vi "Configure VIs for Development.vi"   [LabVIEW 2017]
types:
  T1 = cluster{"Status Message":refnum<data-value>, "Progress":refnum<data-value>, "Stop":refnum<data-value>}
  T2 = enum16{"Share clones between instances", "Preallocate clone for each instance"}
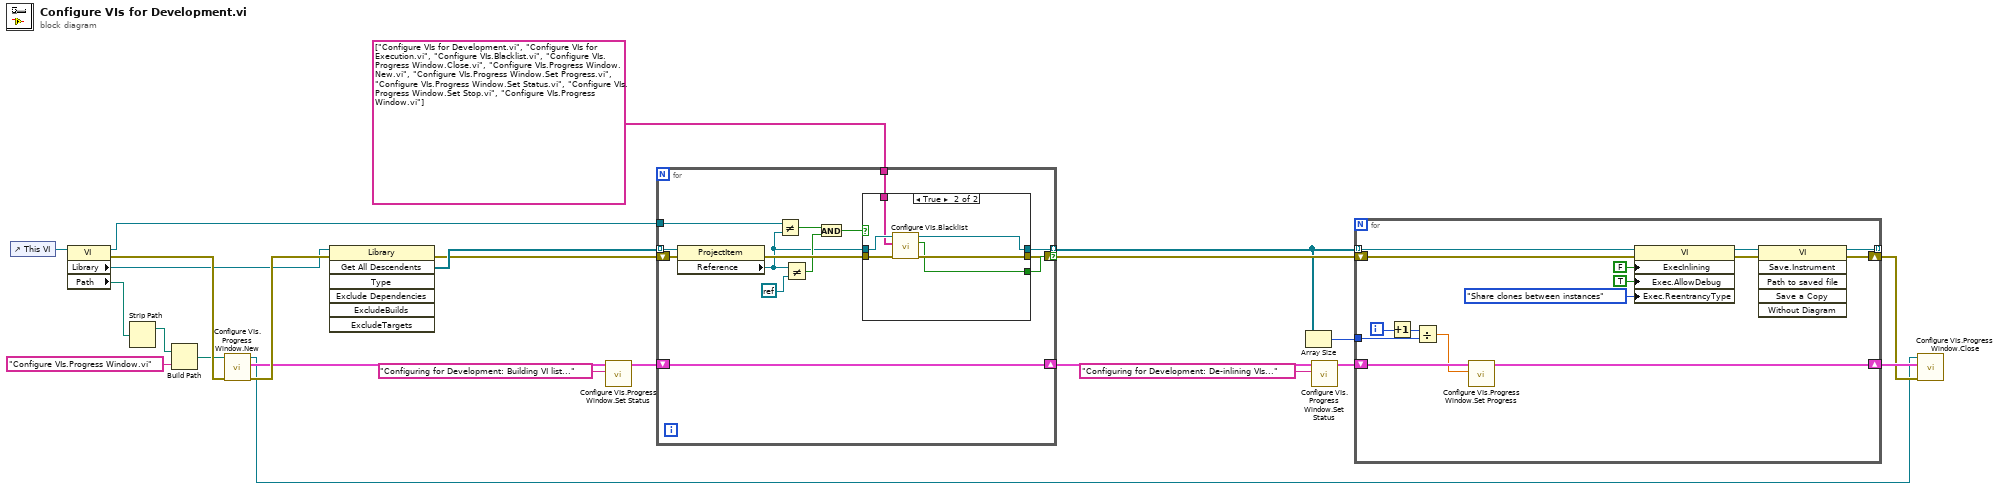
[diagram p0: block diagram]
diagram:
  n1 = control-ref of="This VI"() -> (w24:refnum<vi>)
  n2 = property class="VI"(reference=w24) -> (reference out=w23:refnum<vi>, error out=w17:errorcluster, "Library"=w14:refnum<vi>, "Path"=w18:path)  [unwired: 1 in]
  n3 = Strip Path(path=w18) -> (stripped path=w20:path)  [unwired: 1 out]
  n4 = Build Path(base path=w20, name or relative path="Configure VIs.Progress Window.vi") -> (appended path=w15:path)
  n5 = call "Configure VIs.Progress Window.New.vi"("error in (no error)"=w17, "VI path"=w15) -> ("error out"=w16:errorcluster, "DVRs"=w13:T1, "VI refnum"=w2:refnum<vi>)  [unwired: 7 in]
  n6 = invoke class="Library" method="Get All Descendents"(reference=w14, error in=w16) -> (error out=w7:errorcluster, "All Descendents"=w21:refnum<vi>[])  [unwired: 5 in, 5 out]
  n7 = call "Configure VIs.Progress Window.Set Status.vi"("Status Message"="Configuring for Development: Building VI list..." ("data value"), "DVRs in"=w13) -> ("DVRs out"=w12:T1)  [unwired: 8 in, 1 out]
  n8 = for {
    tunnel: w21 -> [w38] mode=indexing
    tunnel: [w37] -> w6 mode=indexing if=w36
    tunnel: w23 -> [w34]
    shift-right: [w32] -> w22
    shift-left: w7 -> [w31]
    shift-right: [w26] -> w10
    shift-left: w12 -> [w26]
    tunnel: string[] ["Configure VIs for Development.vi", "Configure VIs for Execution.vi", "Configure VIs.Blacklist.vi", "Configure VIs.Progress Window.Close.vi", "Configure VIs.Progress Window.New.vi", "Configure VIs.Progress Window.Set Progress.vi", "Configure VIs.Progress Window.Set Status.vi", "Configure VIs.Progress Window.Set Stop.vi", "Configure VIs.Progress Window.vi"] ("Blacklist VIs") -> [w25]
    n9 = property class="ProjectItem"(reference=w38, error in=w31) -> (error out=w30:errorcluster, "Reference"=w27:refnum<vi>)  [unwired: 1 out]
    n10 = Not Equal?(x=w34, y=w27) -> (x != y?=w33:bool)
    n11 = Not Equal?(x=w27, y=refnum<k0> refnum) -> (x != y?=w29:bool)
    n12 = And(x=w33, y=w29) -> (x .and. y?=w28:bool)
    n13 = case shown="True" w28 {
      selector: w28 -> [w40 _]
      tunnel: [w41 w45] -> w37
      tunnel: [w40 w42] -> w36
      tunnel: w27 -> [w41 w44]
      tunnel: [w39 w46] -> w32
      tunnel: w30 -> [w39 w47]
      tunnel: w25 -> [_ w43]
      frame False {
      }
      frame True {
        n14 = call "Configure VIs.Blacklist.vi"("error in (no error)"=w47, "Blacklist VIs"=w43, "VI reference in"=w44) -> ("error out"=w46:errorcluster, "valid?"=w42:bool, "VI reference out"=w45:refnum<vi>)  [unwired: 6 in]
      }
    }
  }
  n15 = Array Size(array=w6) -> (size(s)=w5:i32)
  n16 = call "Configure VIs.Progress Window.Set Status.vi"("Status Message"="Configuring for Development: De-inlining VIs..." ("data value"), "DVRs in"=w10) -> ("DVRs out"=w9:T1)  [unwired: 8 in, 1 out]
  n17 = for {
    tunnel: w6 -> [w62] mode=indexing
    tunnel: [w55] -> _ mode=indexing
    shift-right: [w54] -> w3
    shift-left: w22 -> [w61]
    shift-right: [w48] -> w4
    shift-left: w9 -> [w50]
    tunnel: w5 -> [w52]
    i -> [w51]
    n18 = Increment(x=w51) -> (x+1=w53:i32)
    n19 = Divide(x=w53, y=w52) -> (x/y=w49:dbl)
    n20 = call "Configure VIs.Progress Window.Set Progress.vi"("Progress"=w49, "DVRs in"=w50) -> ("DVRs out"=w48:T1)  [unwired: 8 in, 1 out]
    n21 = property class="VI"(reference=w62, error in=w61, "ExecInlining"=FALSE ("Execution:Inline SubVI"), "Exec.AllowDebug"=TRUE ("Execution:Allow Debugging"), "Exec.ReentrancyType"=T2."Share clones between instances" ("Execution:Reentrancy Type")) -> (reference out=w56:refnum<vi>, error out=w57:errorcluster)
    n22 = invoke class="VI" method="Save.Instrument"(reference=w56, error in=w57) -> (reference out=w55:refnum<vi>, error out=w54:errorcluster)  [unwired: 4 in, 4 out]
  }
  n23 = call "Configure VIs.Progress Window.Close.vi"("error in (no error)"=w3, "DVRs in"=w4, "VI refnum"=w2) -> ()  [unwired: 8 in, 1 out]
